vi "SetIntTime.vi"(3 "error in":errorcluster, 4 "Integration Time":i32, 5 "SpectRef In":T1) -> (0 "error out":errorcluster, 2 "SpectRef Out":T1)   [LabVIEW 2012]
uses:
  Controls/USB4000_Data.ctl
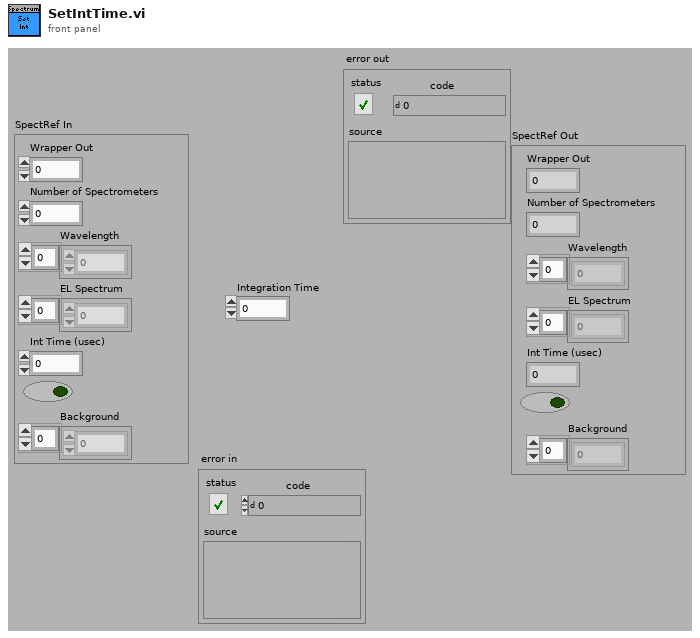
[diagram p1: front panel]
types:
  T1 = typedef "USB4000_Data.ctl" = cluster{"Wrapper Out":u32, "Number of Spectrometers":i32, "Wavelength":dbl[], "EL Spectrum":dbl[], "Int Time (usec)":i32, bool, "Background":dbl[]}
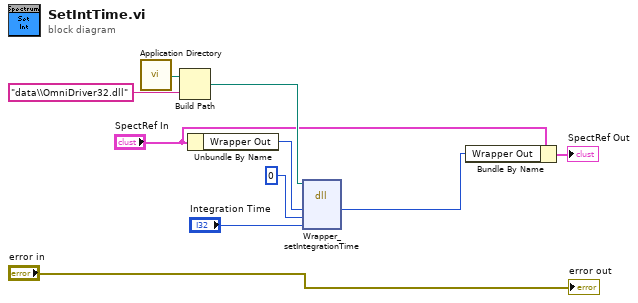
[diagram p0: block diagram]
diagram:
  n1 = call <vilib>:"Application Directory.vi"() -> ("Application Directory"=w9:path)
  n2 = Build Path(base path=w9, name or relative path="data\\OmniDriver32.dll") -> (appended path=w7:path)
  n3 = Unbundle By Name("SpectRef In") -> ("Wrapper Out"=w4:u32)
  n4 = dll-call lib="D:/Software Development/EPI Development/BurnIn Testing/Instruments/Drivers/Ocean Optics/OOI_HOME/OmniDriver32.dll" fn="Wrapper_setIntegrationTime" label="Wrapper.setIntegrationTime"(path in=w7, "Wrapper"=w4, "Index"=0, "Integration Time"="Integration Time") -> ("Wrapper"=w6:u32)  [unwired: 4 in, 3 out]
  n5 = Bundle By Name(cluster="SpectRef In", "Wrapper Out"=w6) -> (→"SpectRef Out":T1)
  "error out" <- "error in"
